vi "GetAMIRequest.vi"() -> (3 "Request":u8[](array[numeric]))   [LabVIEW 2015]
uses:
  <instrlib>/Samwontech TEMP2xxx/Samwontech TEMP2xxx.lvlib
panel:
  out "Request":string
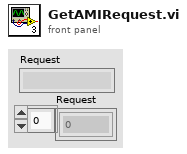
[diagram p1: front panel]
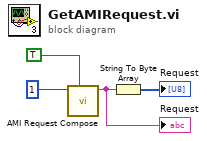
[diagram p0: block diagram]
diagram:
  n1 = call <instrlib>:"AMI Request Compose.vi"("Checksum used"=TRUE, "Address"=u8 1) -> ("Request"=w2:string)  [unwired: 8 in, 1 out]
  "Request" <- w2
  n2 = String To Byte Array(string=w2) -> (unsigned byte array=→"Request":u8[])
